vi "Read Waveform Measurement.vi"   [LabVIEW 2015, in "Tektronix 7000 Series.lvlib"]
doc: "Initiates an acquisition on the channels that you enable with the Configure Channel VI. This VI then waits for the acquisition to complete, obtains a waveform measurement on the channels you specify, and returns the measurement value."
uses:
  <instrlib>/Tektronix 7000 Series/Tektronix 7000 Series.lvlib
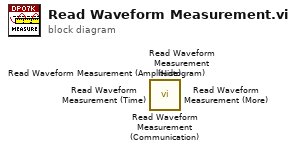
[diagram p0: block diagram]
diagram:
  n1 = call <instrlib>:"Read Waveform Measurement (Communication).vi"() -> ()  [unwired: 13 in, 3 out]
  n2 = call <instrlib>:"Read Waveform Measurement (Histogram).vi"() -> ()  [unwired: 13 in, 3 out]
  n3 = call <instrlib>:"Read Waveform Measurement (Time).vi"() -> ()  [unwired: 13 in, 3 out]
  n4 = call <instrlib>:"Read Waveform Measurement (More).vi"() -> ()  [unwired: 13 in, 3 out]
  n5 = call <instrlib>:"Read Waveform Measurement (Amplitude).vi"() -> ()  [unwired: 13 in, 3 out]
